vi "Get_Port_status.vi"(8 "error in (no error)":errorcluster, 10 "CH":i32, 11 "NXP in":refnum<class "NXP.lvclass">) -> (0 "error out":errorcluster, 1 "Expected Response":string, 2 "Command to Send":string, 3 "NXP out":refnum<class "NXP.lvclass">)   [LabVIEW 2020, in "NXP.lvclass"]
uses:
  NXP.lvclass
  Abstract/Serial Device/Combo Box Comandos.ctl
  Abstract/Serial Device/Combo Box Devices.ctl
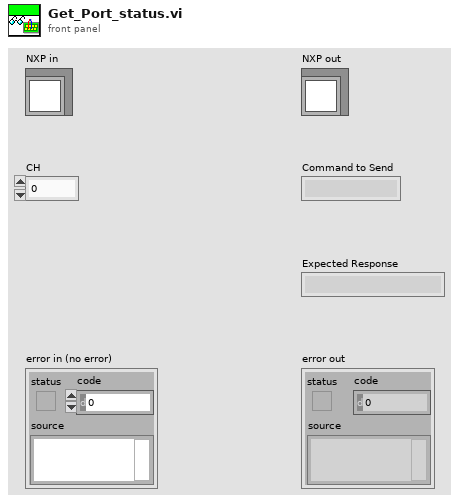
[diagram p1: front panel]
types:
  T1 = typedef "Combo Box Devices.ctl" = string
  T2 = typedef "Combo Box Comandos.ctl" = string
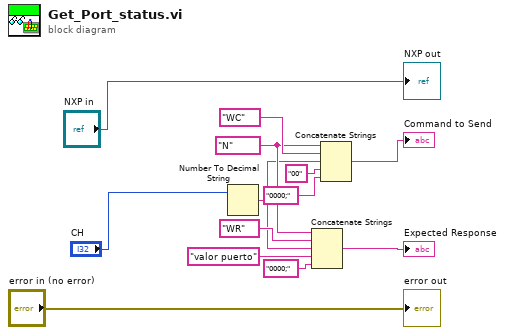
[diagram p0: block diagram]
diagram:
  w12 = T1 "N" ("Serial Devide Brand")
  n1 = Number To Decimal String(number="CH") -> (decimal integer string=w10:string)  [unwired: 1 in]
  n2 = Concatenate Strings(w12, T2 "WR" ("Respuesta"), w10, "valor puerto" ("string"), "0000;" ("string")) -> (→"Expected Response":string)
  n3 = Concatenate Strings(w12, T2 "WC" ("Command"), w10, "00" ("string"), "0000;" ("string")) -> (→"Command to Send":string)
  "error out" <- "error in (no error)"
  "NXP out" <- "NXP in"
